vi "Configure.vi"(8 "error in (no error)":errorcluster, 11 "configuration in":refnum<class "statemachine.lvclass">) -> (0 "error out":errorcluster, 3 "configuration out":refnum<class "statemachine.lvclass">)   [LabVIEW 2020, in "eos.lvlib" / "statemachine.lvclass"]
uses:
  statemachine.lvclass
  interfaces/configuration/configurable.lvclass
  interfaces/initialization/initializable.lvclass
  C:/Projects/LVOS/EngineeringOS/source/interfaces/initialization/initializable.lvclass
  C:/Projects/LVOS/EngineeringOS/source/interfaces/state/state.lvclass
  C:/Projects/LVOS/EngineeringOS/source/interfaces/configuration/configurable.lvclass
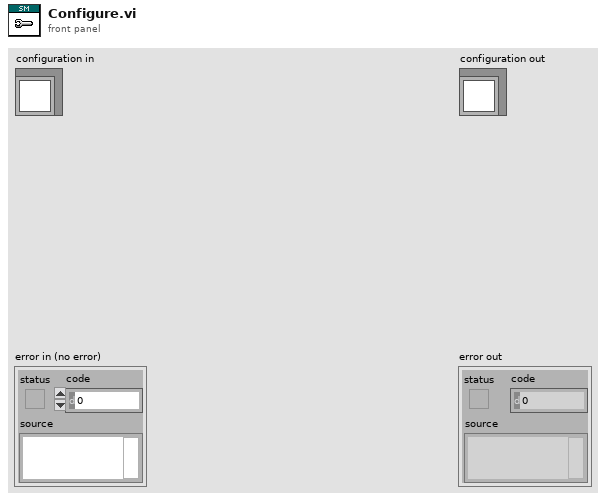
[diagram p1: front panel]
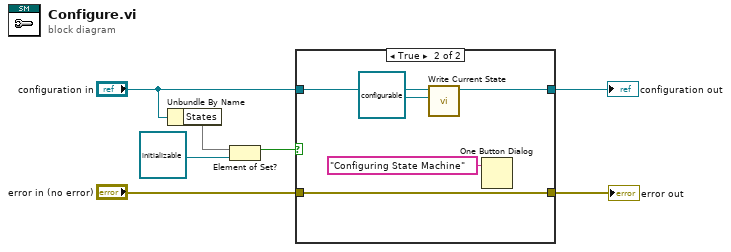
[diagram p0: block diagram]
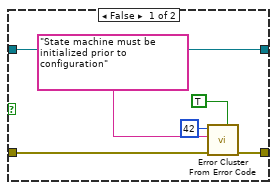
[diagram p2: hidden frame]
diagram:
  n1 = Unbundle By Name("configuration in") -> ("States"=w3:set{refnum<class "state.lvclass">})
  n2 = Element of Set?(10:refnum<class "initializable.lvclass"> refnum ("eos.lvlib:initializable.lvclass"), 11:w3) -> (3:w1:bool)
  n3 = case shown="True" w1 {
    tunnel: [w13 w18] -> w4
    tunnel: "error in (no error)" -> [w12 w18]
    tunnel: "configuration in" -> [w8 w16]
    tunnel: [w8 w17] -> w5
    frame False {
      n4 = call <vilib>:"Error Cluster From Error Code.vi"("is warning? (False)"=TRUE, "error in (no error)"=w12, "error message (\"\")"="State machine must be initialized prior to configuration" ("error message (\"\")"), "error code (0)"=42) -> ("error out"=w13:errorcluster)  [unwired: 5 in]
    }
    frame True {
      n5 = call "Write Current State.vi"("Current State"=refnum<class "configurable.lvclass"> refnum ("eos.lvlib:configurable.lvclass"), "statemachine in"=w16) -> ("statemachine out"=w17:refnum<class "statemachine.lvclass">)  [unwired: 9 in]
      n6 = One Button Dialog(message="Configuring State Machine") -> ()  [unwired: 1 in, 1 out]
    }
  }
  "error out" <- w4
  "configuration out" <- w5
